vi "HFRR ADV v01.vi"() -> ()   [LabVIEW 2025] (continued)
                w439 = T19."Enabled" ("Disabled")
                n341 = property on="Auto Start Test" class="Bool (strict)"("DisabledEnum"=w439, "TipStrip"=w438) -> ()  [unwired: 2 in, 2 out]
                n342 = property on="RUN" class="Bool (strict)"("DisabledEnum"=w439, "TipStrip"=w438) -> ()  [unwired: 2 in, 2 out]
              }
              frame False {
                w440 = "Enter File Name to Start Test" ("Tip Strip")
                w441 = T19."Disabled and Grayed Out" ("Disabled")
                n343 = property on="Auto Start Test" class="Bool (strict)"("DisabledEnum"=w441, "TipStrip"=w440) -> ()  [unwired: 2 in, 2 out]
                n344 = property on="RUN" class="Bool (strict)"("DisabledEnum"=w441, "TipStrip"=w440) -> ()  [unwired: 2 in, 2 out]
              }
            }
          }
          frame True {
            w442 = "" ("Tip Strip")
            w443 = T19."Enabled" ("Disabled")
            n345 = property on="Auto Start Test" class="Bool (strict)"("DisabledEnum"=w443, "TipStrip"=w442) -> ()  [unwired: 2 in, 2 out]
            n346 = property on="RUN" class="Bool (strict)"("DisabledEnum"=w443, "TipStrip"=w442) -> ()  [unwired: 2 in, 2 out]
          }
        }
      }
      event "RUN": Value Change {
        n347 = event-data() -> ()  [unwired: 1 in, 6 out]
        n348 = local read "RUN"() -> (w445:bool)
        n349 = case shown="False" w445 {
          frame False {
            n350 = flat-sequence {
              frame #0 {
                n351 = local write "START TEMP"(FALSE ("START TEMP")) -> ()
              }
              frame #1 {
                n352 = Wait (ms)(milliseconds to wait=u32 1500) -> ()  [unwired: 1 out]
              }
              frame #2 {
                n353 = local write "Humidity 2"(TRUE ("Humidity")) -> ()
              }
              frame #3 {
                n354 = local write "Due Write"("VC;0") -> ()
              }
              frame #4 {
                n355 = Wait (ms)(milliseconds to wait=u32 1500) -> ()  [unwired: 1 out]
              }
              frame #5 {
                w455 = T19."Enabled" ("Disabled")
                (unwired) T25."Imaging" ("Main Dashboard Buttons")
                (unwired) T21."Adv Scar" ("Main Tab")
                w457 = "" ("FILE")
                n356 = local write "measured_stroke"(0.0 ("measured_stroke")) -> ()
                n357 = local write "Due Write"("VC;0") -> ()
                n358 = local write "FILE"(w457) -> ()
                n359 = local write "Batch Ref Num :"(w457) -> ()
                n360 = local write "Fuel Discription :"(w457) -> ()
                n361 = local write "Main Tab"(T4."Adv Scar" ("Main Tab")) -> ()
                n362 = local write "Remarks :"(w457) -> ()
                n363 = local write "Main Dashboard Buttons"(T1."Imaging" ("Main Dashboard Buttons")) -> ()
                n364 = local write "TEST FILE NAM,E SAVED"(FALSE ("TEST FILE NAM,E SAVED")) -> ()
                n365 = property on="Stroke ( mm )" class="WFChart (strict)"("History Data"=cluster{"y":dbl, dbl, "y":dbl}[] []) -> ()  [unwired: 2 in, 2 out]
                n366 = property on="Auto Start Test" class="Bool (strict)"("Visible"=TRUE) -> ()  [unwired: 2 in, 2 out]
                n367 = property on="FRICVALZ 2" class="Bool (strict)"("DisabledEnum"=w455) -> ()  [unwired: 2 in, 2 out]
                n368 = property on="FRICVALZ 4" class="Bool (strict)"("DisabledEnum"=w455) -> ()  [unwired: 2 in, 2 out]
                n369 = property on="FRICVALZ 3" class="Bool (strict)"("DisabledEnum"=w455) -> ()  [unwired: 2 in, 2 out]
              }
            }
          }
          frame True {
            n370 = stacked-sequence {
              frame #0 {
                n371 = local write "FRICVALZ 4"(TRUE ("FRICVALZ 4")) -> ()
                n372 = local write "Due Write"("DAC;200") -> ()
              }
              frame #1 {
              }
              frame #2 {
              }
              frame #3 {
                n373 = Wait (ms)(milliseconds to wait=u32 1000) -> ()  [unwired: 1 out]
              }
              frame #4 {
                n374 = local write "Due Write"("VC;1") -> ()
              }
              frame #5 {
                n375 = Wait (ms)(milliseconds to wait=u32 1000) -> ()  [unwired: 1 out]
              }
              frame #6 {
                n376 = local write "Due Write"("VC;1") -> ()
              }
              frame #7 {
                n377 = Wait (ms)(milliseconds to wait=u32 1500) -> ()  [unwired: 1 out]
              }
              frame #8 {
                w468 = T19."Disabled" ("Disabled")
                n378 = property on="Auto Start Test" class="Bool (strict)"("Visible"=FALSE) -> ()  [unwired: 2 in, 2 out]
                n379 = local write "START TEMP"(TRUE ("START TEMP")) -> ()
                n380 = property on="FRICVALZ 2" class="Bool (strict)"("DisabledEnum"=w468) -> ()  [unwired: 2 in, 2 out]
                n381 = property on="FRICVALZ 4" class="Bool (strict)"("DisabledEnum"=w468) -> ()  [unwired: 2 in, 2 out]
                n382 = property on="FRICVALZ 3" class="Bool (strict)"("DisabledEnum"=w468) -> ()  [unwired: 2 in, 2 out]
              }
            }
          }
        }
      }
      event "run test Calibration": Value Change {
        n383 = event-data() -> ()  [unwired: 1 in, 6 out]
        n384 = local read "run test Calibration"() -> (w470:bool)
        n385 = case shown="False" w470 {
          frame False {
            n386 = flat-sequence {
              frame #0 {
                n387 = local write "START TEMP"(FALSE ("START TEMP")) -> ()
              }
              frame #1 {
                n388 = Wait (ms)(milliseconds to wait=u32 1500) -> ()  [unwired: 1 out]
              }
              frame #2 {
              }
              frame #3 {
                n389 = local write "Due Write"("VC;0") -> ()
              }
              frame #4 {
                n390 = Wait (ms)(milliseconds to wait=u32 1500) -> ()  [unwired: 1 out]
              }
              frame #5 {
                n391 = local write "Due Write"("VC;0") -> ()
                n392 = property on="Tab Control 6" class="TabCtl (strict)"("Visible"=FALSE) -> ()  [unwired: 2 in, 2 out]
                n393 = local write "Friction Force Calibration Result Tab"(enum32{"Calibration Results", "Page 2"}."Calibration Results" ("Friction Force Calibration Result Tab")) -> ()
                n394 = property on="Friction Force Calibration Result Tab" class="TabCtl (strict)"("Visible"=TRUE) -> ()  [unwired: 2 in, 2 out]
              }
            }
          }
          frame True {
            n395 = flat-sequence {
              frame #0 {
                n396 = local write "Due Write"("VC;1") -> ()
              }
              frame #1 {
                n397 = Wait (ms)(milliseconds to wait=u32 1000) -> ()  [unwired: 1 out]
              }
              frame #2 {
                n398 = local write "Due Write"("VC;1") -> ()
              }
              frame #3 {
                n399 = Wait (ms)(milliseconds to wait=u32 2000) -> ()  [unwired: 1 out]
              }
              frame #4 {
                n400 = local write "START TEMP"(TRUE ("START TEMP")) -> ()
                n401 = property on="Tab Control 6" class="TabCtl (strict)"("Visible"=TRUE) -> ()  [unwired: 2 in, 2 out]
                n402 = local write "Friction Force Calibration Result Tab"(enum32{"Calibration Results", "Page 2"}."Calibration Results" ("Friction Force Calibration Result Tab")) -> ()
              }
            }
          }
        }
      }
      event "Auto": Value Change {
        n403 = event-data() -> ()  [unwired: 1 in, 6 out]
        n404 = stacked-sequence {
          frame #0 {
            n405 = local write "FILE"("") -> ()
          }
          frame #1 {
            n406 = Get Date/Time In Seconds() -> (seconds since 1Jan1904=w491:timestamp)
            n407 = Format Into String(format string="%<%m/%d/%Y %I:%M:%S %p>T", w491) -> (resulting string=w490:string)  [unwired: 2 in, 1 out]
            n408 = local write "FILE"(w490) -> ()
          }
        }
        n409 = local read "Auto"() -> (w488:bool)
        n410 = Not(x=w488) -> (.not. x?=w487:bool)
        n411 = local write "Auto"(w487) -> ()
      }
      event "Auto Start Temp": Value Change {
        n412 = event-data() -> ()  [unwired: 1 in, 6 out]
        n413 = local read "Auto Start Test"() -> (w494:bool)
        n414 = case shown="False" w494 {
          frame False {
            n415 = stacked-sequence {
              frame #0 {
                n416 = local write "START TEMP"(FALSE ("START TEMP")) -> ()
              }
              frame #1 {
                n417 = Wait (ms)(milliseconds to wait=u32 2000) -> ()  [unwired: 1 out]
              }
              frame #2 {
                n418 = local write "Due Write"("VC;0") -> ()
              }
              frame #3 {
                n419 = Wait (ms)(milliseconds to wait=u32 2000) -> ()  [unwired: 1 out]
              }
              frame #4 {
                w505 = T19."Enabled" ("Disabled")
                (unwired) T25."Imaging" ("Main Dashboard Buttons")
                w506 = "" ("FILE")
                n420 = local write "Main Tab"(T4."Adv Scar" ("Main Tab")) -> ()
                n421 = local write "measured_stroke"(0.0 ("measured_stroke")) -> ()
                n422 = local write "Main Dashboard Buttons"(T1."Imaging" ("Main Dashboard Buttons")) -> ()
                n423 = property on="RUN" class="Bool (strict)"("Visible"=TRUE) -> ()  [unwired: 2 in, 2 out]
                n424 = local write "Due Write"("VC;0") -> ()
                n425 = local write "Humidity 2"(TRUE ("Humidity")) -> ()
                n426 = local write "TEST FILE NAM,E SAVED"(FALSE ("TEST FILE NAM,E SAVED")) -> ()
                n427 = local write "Fuel Discription :"(w506) -> ()
                n428 = local write "Batch Ref Num :"(w506) -> ()
                n429 = local write "Remarks :"(w506) -> ()
                n430 = local write "FILE"(w506) -> ()
                n431 = property on="FRICVALZ 2" class="Bool (strict)"("DisabledEnum"=w505) -> ()  [unwired: 2 in, 2 out]
                n432 = property on="FRICVALZ 4" class="Bool (strict)"("DisabledEnum"=w505) -> ()  [unwired: 2 in, 2 out]
                n433 = property on="FRICVALZ 3" class="Bool (strict)"("DisabledEnum"=w505) -> ()  [unwired: 2 in, 2 out]
              }
            }
          }
          frame True {
            n434 = stacked-sequence {
              frame #0 {
                n435 = local write "Due Write"("DAC;200") -> ()
              }
              frame #1 {
                n436 = Wait (ms)(milliseconds to wait=u32 1000) -> ()  [unwired: 1 out]
              }
              frame #2 {
              }
              frame #3 {
              }
              frame #4 {
                n437 = local write "Due Write"("VC;1") -> ()
              }
              frame #5 {
                n438 = Wait (ms)(milliseconds to wait=u32 1000) -> ()  [unwired: 1 out]
              }
              frame #6 {
                n439 = local write "Due Write"("VC;1") -> ()
              }
              frame #7 {
                n440 = Wait (ms)(milliseconds to wait=u32 1500) -> ()  [unwired: 1 out]
              }
              frame #8 {
                w515 = T19."Disabled" ("Disabled")
                n441 = property on="RUN" class="Bool (strict)"("Visible"=FALSE) -> ()  [unwired: 2 in, 2 out]
                n442 = property on="FRICVALZ 2" class="Bool (strict)"("DisabledEnum"=w515) -> ()  [unwired: 2 in, 2 out]
                n443 = property on="FRICVALZ 4" class="Bool (strict)"("DisabledEnum"=w515) -> ()  [unwired: 2 in, 2 out]
                n444 = property on="FRICVALZ 3" class="Bool (strict)"("DisabledEnum"=w515) -> ()  [unwired: 2 in, 2 out]
                "START TEMP" <- TRUE
              }
            }
          }
        }
      }
      event "FILE", "USERNAME", "USER ID": Mouse Enter {
        n445 = event-data() -> ()  [unwired: 1 in, 4 out]
        n446 = dll-call lib="kernel32.dll" fn="Wow64DisableWow64FsRedirection"("OldValue"=0) -> (error out=w522:errorcluster, "OldValue"=w520:i32)  [unwired: 4 in, 1 out]
        n447 = call <vilib>:"System Exec.vi"("run minimized? (F)"=TRUE, "error in (no error)"=w522, "command line"="C:\\Program Files\\Common Files\\Microsoft Shared\\Ink\\TabTip.exe") -> ("error out"=w521:errorcluster)  [unwired: 5 in, 3 out]
        n448 = dll-call lib="kernel32.dll" fn="Wow64EnableWow64FsRedirection"(error in=w521, "OldValue"=w520) -> ()  [unwired: 4 in, 2 out]
      }
      event "EDIT": Value Change {
        n449 = event-data() -> ()  [unwired: 1 in, 6 out]
        n450 = local read "EDIT"() -> (w523:bool)
        n451 = case shown="False" w523 {
          frame False {
            n452 = control-ref of="This VI"() -> (w540:refnum<vi>)
            n453 = property class="VI"(reference=w540) -> (reference out=w531:refnum<vi>, error out=w535:errorcluster, "Panel"=w539:refnum<vi>)  [unwired: 1 in]
            n454 = property class="Pnl"(reference=w539, error in=w535) -> (reference out=w533:refnum<vi>, error out=w536:errorcluster, "Panes[]"=w538:refnum<vi>[])
            n455 = for {
              tunnel: w538 -> [w546] mode=indexing
              tunnel: T24."Always Off" ("Horizontal Scrollbar Visibility") -> [w545]
              tunnel: w536 -> [w542]
              tunnel: [w541] -> w534
              n456 = property class="Pane"(reference=w546, error in=w542, "HorizScrollbarVisibility"=w545) -> (reference out=w543:refnum<vi>, error out=w544:errorcluster)
              n457 = Close Reference(reference=w543, error in (no error)=w544) -> (error out=w541:errorcluster)
            }
            n458 = Close Reference(reference=w533, error in (no error)=w534) -> (error out=w532:errorcluster)
            n459 = Close Reference(reference=w531, error in (no error)=w532) -> (error out=w526:errorcluster)
            "error out 7" <- w526
            n460 = call <vilib>:"Clear Errors.vi"("error in (no error)"=w526) -> ("error out"=w525:errorcluster)  [unwired: 5 in, 1 out]
            n461 = local write "Service Password enable"(FALSE ("Service Password enable")) -> ()
            n462 = call <userlib>:"Fit VI window to Largest Dec.vi"("error in (no error)"=w525, "border spacing (2 px)"=1) -> ("error out"=w530:errorcluster, "dup VI Ref"=w528:refnum<vi>)  [unwired: 4 in]
            n463 = invoke on="Invoke Node" class="VI" method="FP.Run-Time Position.Maximized"(reference=w528, error in=w530) -> (error out=w529:errorcluster)  [unwired: 2 in, 3 out]
            n464 = call <vilib>:"Clear Errors.vi"("error in (no error)"=w529) -> ()  [unwired: 5 in, 2 out]
          }
          frame True {
          }
        }
      }
      event "Heater Button": Value Change {
        n465 = event-data() -> ()  [unwired: 1 in, 6 out]
        n466 = local read "Heater Button"() -> (w547:bool)
        n467 = case shown="True" w547 {
          frame True {
            n468 = stacked-sequence {
              frame #0 {
                n469 = Wait (ms)(milliseconds to wait=u32 1500) -> ()  [unwired: 1 out]
              }
              frame #1 {
                n470 = local read "Set Temp"() -> (w549:dbl)
                n471 = Number To Fractional String(number=w549, precision (6)=i16 2) -> (F-format string=w552:string)  [unwired: 2 in]
                n472 = Concatenate Strings("ST;" ("Command"), w552) -> (w551:string)
                n473 = local write "Due Write"(w551) -> ()
              }
              frame #2 {
                n474 = Wait (ms)(milliseconds to wait=u32 1500) -> ()  [unwired: 1 out]
              }
              frame #3 {
                n475 = local write "Due Write"("HE;1" ("Command")) -> ()
              }
              frame #4 {
                n476 = Wait (ms)(milliseconds to wait=u32 1500) -> ()  [unwired: 1 out]
              }
              frame #5 {
                n477 = stacked-sequence {
                  frame #0 {
                    n478 = Wait (ms)(milliseconds to wait=u32 1500) -> ()  [unwired: 1 out]
                  }
                  frame #1 {
                    n479 = local read "Set Temp"() -> (w558:dbl)
                    n480 = Number To Fractional String(number=w558, precision (6)=i16 2) -> (F-format string=w561:string)  [unwired: 2 in]
                    n481 = Concatenate Strings("ST;" ("Command"), w561) -> (w560:string)
                    n482 = local write "Due Write"(w560) -> ()
                  }
                  frame #2 {
                    n483 = Wait (ms)(milliseconds to wait=u32 1500) -> ()  [unwired: 1 out]
                  }
                  frame #3 {
                    n484 = local write "Due Write"("HE;1" ("Command")) -> ()
                  }
                  frame #4 {
                    n485 = Wait (ms)(milliseconds to wait=u32 1500) -> ()  [unwired: 1 out]
                  }
                }
              }
            }
          }
          frame False {
            n486 = stacked-sequence {
              frame #0 {
                n487 = Wait (ms)(milliseconds to wait=u32 1500) -> ()  [unwired: 1 out]
              }
              frame #1 {
                n488 = Concatenate Strings("ST;" ("Command"), "0" ("string")) -> (w568:string)
                n489 = local write "Due Write"(w568) -> ()
              }
              frame #2 {
                n490 = Wait (ms)(milliseconds to wait=u32 1500) -> ()  [unwired: 1 out]
              }
              frame #3 {
                n491 = local write "Due Write"("HE;0" ("Command")) -> ()
              }
              frame #4 {
                n492 = Wait (ms)(milliseconds to wait=u32 1500) -> ()  [unwired: 1 out]
              }
            }
          }
        }
      }
      event "Headen Service Button": Value Change {
        n493 = event-data() -> ()  [unwired: 1 in, 6 out]
        n494 = local read "Headen Service Button"() -> (w573:bool)
        n495 = case shown="True" w573 {
          frame False {
            n496 = property on="Password 3" class="Clust (strict)"("Visible"=FALSE) -> ()  [unwired: 2 in, 2 out]
            n497 = property on="Service Password Log" class="Str"("Visible"=FALSE) -> ()  [unwired: 2 in, 2 out]
          }
          frame True {
            n498 = flat-sequence {
              tunnel: [w579] -> w576
              tunnel: w576 -> [w580]
              frame #0 {
                n499 = property on="Password 3" class="Clust (strict)"("Visible"=TRUE) -> ()  [unwired: 2 in, 2 out]
                n500 = property on="Service Password Log" class="Str"("Visible"=TRUE) -> ()  [unwired: 2 in, 2 out]
              }
              frame #1 {
                n501 = call "DIALOG BOX HFRR ADV.vi"() -> ("Continue"=w579:bool)  [unwired: 8 in, 2 out]
              }
              frame #2 {
                n502 = case shown="True" w580 {
                  frame True {
                    n503 = property on="Password 3" class="Clust (strict)"("Visible"=TRUE) -> ()  [unwired: 2 in, 2 out]
                    n504 = property on="Service Password Log" class="Str"("Visible"=TRUE) -> ()  [unwired: 2 in, 2 out]
                  }
                  frame False {
                    n505 = property on="Password 3" class="Clust (strict)"("Visible"=FALSE) -> ()  [unwired: 2 in, 2 out]
                    n506 = property on="Service Password Log" class="Str"("Visible"=FALSE) -> ()  [unwired: 2 in, 2 out]
                  }
                }
              }
            }
          }
        }
      }
      event "Password 3.Service Password": Value Change {
        n507 = event-data() -> ()  [unwired: 1 in, 6 out]
        n508 = Unbundle By Name("Password 3") -> ("Service Password"=w587:string)
        n509 = call <vilib>:"Trim Whitespace.vi"("string"=w587) -> ("trimmed string"=w585:string)  [unwired: 1 in]
        n510 = Equal?(x=w585, y="Service@123") -> (x = y?=w586:bool)
        n511 = case shown="True" w586 {
          selector: w586 -> [w591 w594]
          frame False {
            w590 = FALSE
            n512 = local write "Service Password enable"(w591) -> ()
            n513 = property on="Service Password Log" class="Str"("Visible"=TRUE) -> ()  [unwired: 2 in, 2 out]
            n514 = property on="Service Left" class="Bool (strict)"("Visible"=w590) -> ()  [unwired: 2 in, 2 out]
            n515 = property on="Service Right" class="Bool (strict)"("Visible"=w590) -> ()  [unwired: 2 in, 2 out]
            n516 = property on="Service Bottom" class="Bool (strict)"("Visible"=w590) -> ()  [unwired: 2 in, 2 out]
          }
          frame True {
            w593 = TRUE
            n517 = property on="Service Password Log" class="Str"("Visible"=FALSE) -> ()  [unwired: 2 in, 2 out]
            n518 = property on="Service Left" class="Bool (strict)"("Visible"=w593) -> ()  [unwired: 2 in, 2 out]
            n519 = property on="Service Right" class="Bool (strict)"("Visible"=w593) -> ()  [unwired: 2 in, 2 out]
            n520 = property on="Service Bottom" class="Bool (strict)"("Visible"=w593) -> ()  [unwired: 2 in, 2 out]
            "Service Password enable" <- w594
          }
        }
      }
      event "Sign In": Value Change {
        w596 = FALSE ("Visible")
        n521 = event-data() -> ()  [unwired: 1 in, 6 out]
        n522 = property on="About" class="Clust (strict)"("Visible"=w596) -> ()  [unwired: 2 in, 2 out]
        n523 = property on="Password 3" class="Clust (strict)"("Visible"=w596) -> ()  [unwired: 2 in, 2 out]
        n524 = property on="Service Password Log" class="Str"("Visible"=FALSE) -> ()  [unwired: 2 in, 2 out]
      }
      event "Info": Value Change {
        n525 = event-data() -> ()  [unwired: 1 in, 6 out]
        n526 = local read "Operating System"() -> (w601:string)
        n527 = local read "Firmware Version"() -> (w602:string)
        n528 = local read "Instrument Serial"() -> (w600:string)
        n529 = local read "Workorder"() -> (w604:string)
        n530 = local write "Info"(FALSE) -> ()
        n531 = local read "Runtime"() -> (w603:string)
        n532 = local read "Version"() -> (w605:string)
        n533 = local read "version"() -> (w606:string)
        n534 = Insert Into Array(array=string[] [], new element #1=w606, new element #2=w605, new element #3=w604, new element #4=w603, new element #5=w602, new element #6=w601, new element #7=w600) -> (w599:string[])  [unwired: 1 in]
        n535 = call "ABOUT SCREEN ADV NEW.vi"("Array"=w599) -> ()  [unwired: 10 in, 1 out]
      }
      event "Calibration": Value Change {
        n536 = event-data() -> ()  [unwired: 1 in, 6 out]
        n537 = local read "Calibration"() -> (w609:bool)
        n538 = case shown="False" w609 {
          frame False {
            n539 = property on="Calibration 2" class="TabCtl (strict)"("Visible"=FALSE) -> ()  [unwired: 2 in, 2 out]
            n540 = local write "Cal Password"("" ("Cal Password")) -> ()
          }
          frame True {
            n541 = property on="Calibration 2" class="TabCtl (strict)"("Visible"=TRUE) -> ()  [unwired: 2 in, 2 out]
            n542 = local write "Cal Password"("" ("Cal Password")) -> ()
          }
        }
        n543 = property on="Wrong Password" class="Str"("Visible"=FALSE) -> ()  [unwired: 2 in, 2 out]
      }
      event "Cal Password": Value Change {
        n544 = event-data() -> ()  [unwired: 1 in, 6 out]
        n545 = local read "Cal Password"() -> (w617:string)
        n546 = call <vilib>:"Trim Whitespace.vi"("string"=w617) -> ("trimmed string"=w616:string)  [unwired: 1 in]
        n547 = Equal?(x=w616, y="Cal@321") -> (x = y?=w614:bool)
        n548 = case shown="True" w614 {
          frame False {
            n549 = property on="Wrong Password" class="Str"("Visible"=TRUE) -> ()  [unwired: 2 in, 2 out]
          }
          frame True {
            n550 = property on="Wrong Password" class="Str"("Visible"=FALSE) -> ()  [unwired: 2 in, 2 out]
            n551 = local write "Main Tab"(T4."About" ("Main Tab")) -> ()
            n552 = local write "Cal Password"("" ("Cal Password")) -> ()
            n553 = local write "Main Dashboard Buttons"(T1."About" ("Main Dashboard Buttons")) -> ()
            n554 = property on="Calibration 2" class="TabCtl (strict)"("Visible"=FALSE) -> ()  [unwired: 2 in, 2 out]
            n555 = local write "Calibration"(FALSE ("Calibration")) -> ()
          }
        }
      }
      event "Calibration Selection": Value Change {
        n556 = event-data() -> ()  [unwired: 1 in, 6 out]
        n557 = local read "Calibration Selection"() -> (w626:T10)
        n558 = case shown="\"Stroke Calibration\"" w626 {
          tunnel: [T9."Stroke" ("Main Calibration Tab") T9."Friction" ("Main Calibration Tab") T9."Main" ("Main Calibration Tab") T9."Temperature" ("Main Calibration Tab")] -> w625
          frame "Stroke Calibration" {
          }
          frame "Friction Force Calibration" {
          }
          frame Default {
          }
          frame "Temperature Calibration" {
          }
        }
        n559 = local write "Main Calibration Tab"(w625) -> ()
      }
      event "Back Stroke": Value Change {
        n560 = event-data() -> ()  [unwired: 1 in, 6 out]
        n561 = local write "Main Stroke Tab"(T11."Step 1" ("Main Stroke Tab")) -> ()
        n562 = local write "Main Calibration Tab"(T9."Main" ("Main Calibration Tab")) -> ()
        n563 = local write "Back Stroke"(FALSE ("Back Stroke")) -> ()
        n564 = local write "Calibration Selection"(T10."Default" ("Calibration Selection")) -> ()
      }
      event "Step 2 Back": Value Change {
        n565 = event-data() -> ()  [unwired: 1 in, 6 out]
        n566 = local write "Main Stroke Tab"(T11."Step 1" ("Main Stroke Tab")) -> ()
        n567 = local write "Step 2 Back"(FALSE ("Back Stroke")) -> ()
        n568 = local write "Calibration Selection"(T10."Default" ("Calibration Selection")) -> ()
      }
      event "Step 3 Back": Value Change {
        n569 = event-data() -> ()  [unwired: 1 in, 6 out]
        n570 = local write "Main Stroke Tab"(T11."Step 2" ("Main Stroke Tab")) -> ()
        n571 = local write "Step 3 Back"(FALSE ("Back Stroke")) -> ()
        n572 = local write "Calibration Selection"(T10."Default" ("Calibration Selection")) -> ()
      }
      event "Step 4 Back": Value Change {
        n573 = event-data() -> ()  [unwired: 1 in, 6 out]
        n574 = local write "Main Stroke Tab"(T11."Step 3" ("Main Stroke Tab")) -> ()
        n575 = local write "Step 4 Back"(FALSE ("Back Stroke")) -> ()
        n576 = local write "Calibration Selection"(T10."Default" ("Calibration Selection")) -> ()
      }
      event "Step 5 Back": Value Change {
        n577 = event-data() -> ()  [unwired: 1 in, 6 out]
        n578 = local write "Main Stroke Tab"(T11."Step 4" ("Main Stroke Tab")) -> ()
        n579 = local write "Step 5 Back"(FALSE ("Back Stroke")) -> ()
        n580 = local write "Calibration Selection"(T10."Default" ("Calibration Selection")) -> ()
      }
      event "Step 6 Back": Value Change {
        n581 = event-data() -> ()  [unwired: 1 in, 6 out]
        n582 = local write "Main Stroke Tab"(T11."Step 5" ("Main Stroke Tab")) -> ()
        n583 = local write "Step 6 Back"(FALSE ("Back Stroke")) -> ()
        n584 = local write "Calibration Selection"(T10."Default" ("Calibration Selection")) -> ()
      }
      event "Back Stroke step 7": Value Change {
        n585 = event-data() -> ()  [unwired: 1 in, 6 out]
        n586 = local write "Main Stroke Tab"(T11."Step 5" ("Main Stroke Tab")) -> ()
        n587 = local write "Back Stroke step 7"(FALSE ("Back Stroke")) -> ()
        n588 = local write "Calibration Selection"(T10."Default" ("Calibration Selection")) -> ()
      }
      event "Back Stroke step 8": Value Change {
        n589 = event-data() -> ()  [unwired: 1 in, 6 out]
        n590 = local write "Main Stroke Tab"(T11."Step 7" ("Main Stroke Tab")) -> ()
        n591 = local write "Back Stroke step 8"(FALSE ("Back Stroke")) -> ()
        n592 = local write "Calibration Selection"(T10."Default" ("Calibration Selection")) -> ()
      }
      event "Back Stroke 8": Value Change {
        n593 = event-data() -> ()  [unwired: 1 in, 6 out]
        n594 = local write "MOVE CARRIAGE TO"(1.0 ("MOVE CARRIAGE TO")) -> ()
        n595 = local write "Main Stroke Tab"(T11."Step 1" ("Main Stroke Tab")) -> ()
        n596 = local write "Calibration Selection"(T10."Default" ("Calibration Selection")) -> ()
        n597 = local write "Back Stroke 8"(FALSE ("Back Stroke 8")) -> ()
      }
      event "Continue Stroke": Value Change {
        n598 = event-data() -> ()  [unwired: 1 in, 6 out]
        n599 = local write "Main Stroke Tab"(T11."Step 2" ("Main Stroke Tab")) -> ()
        n600 = local write "Continue Stroke"(FALSE ("Continue Stroke")) -> ()
      }
      event "Continue Stroke step 2": Value Change {
        n601 = event-data() -> ()  [unwired: 1 in, 6 out]
        n602 = local write "Main Stroke Tab"(T11."Step 3" ("Main Stroke Tab")) -> ()
        n603 = local write "Continue Stroke step 2"(FALSE ("Continue Stroke")) -> ()
      }
      event "Continue Stroke step 3": Value Change {
        n604 = event-data() -> ()  [unwired: 1 in, 6 out]
        n605 = local write "Main Stroke Tab"(T11."Step 4" ("Main Stroke Tab")) -> ()
        n606 = local write "Continue Stroke step 3"(FALSE ("Continue Stroke")) -> ()
      }
      event "Continue Stroke step 4": Value Change {
        n607 = event-data() -> ()  [unwired: 1 in, 6 out]
        n608 = local write "Main Stroke Tab"(T11."Step 5" ("Main Stroke Tab")) -> ()
        n609 = local write "Continue Stroke step 4"(FALSE ("Continue Stroke")) -> ()
      }
      event "Continue Stroke step 5": Value Change {
        n610 = event-data() -> ()  [unwired: 1 in, 6 out]
        n611 = local write "Main Stroke Tab"(T11."Step 7" ("Main Stroke Tab")) -> ()
        n612 = local write "Continue Stroke step 5"(FALSE ("Continue Stroke")) -> ()
      }
      event "Continue Stroke step 6": Value Change {
        n613 = event-data() -> ()  [unwired: 1 in, 6 out]
        n614 = local write "Main Stroke Tab"(T11."Step 7" ("Main Stroke Tab")) -> ()
        n615 = local write "Continue Stroke step 6"(FALSE ("Continue Stroke")) -> ()
      }
      event "Continue Stroke step 7": Value Change {
        w674 = FALSE ("0.2mm")
        n616 = event-data() -> ()  [unwired: 1 in, 6 out]
        n617 = local write "0.4 mm"(w674) -> ()
        n618 = local write "0.6 mm"(w674) -> ()
        n619 = local write "1.0 mm"(w674) -> ()
        n620 = local write "1.2 mm"(w674) -> ()
        n621 = local write "0.2 2"(w674) -> ()
        n622 = local write "0.4 2"(w674) -> ()
        n623 = local write "0.6 2"(w674) -> ()
        n624 = local write "0.8 2"(w674) -> ()
        n625 = local write "1.0 2"(w674) -> ()
        n626 = local write "1.2"(w674) -> ()
        n627 = local write "0.2mm"(w674) -> ()
        n628 = local write "0.8mm"(w674) -> ()
        n629 = local write "Main Stroke Tab"(T11."Step 8" ("Main Stroke Tab")) -> ()
        n630 = local write "Continue Stroke step 7"(FALSE ("Continue Stroke")) -> ()
        n631 = local write "Stroke Test Complete"(T12."Test Progress" ("Stroke Test Complete")) -> ()
        "Position Measurment Temp" <- 4.0 ("Position Measurment Temp")
        "Calibration Tare" <- TRUE ("Calibration Tare")
        "MOVE CARRIAGE TO" <- 1.0 ("MOVE CARRIAGE TO")
      }
      event "Continue Stroke step 8": Value Change {
        n632 = event-data() -> ()  [unwired: 1 in, 6 out]
        n633 = local read "LVDT STROKE  Calibration"() -> (w679:dbl)
        n634 = local read "Position Measurment Temp"() -> (w680:dbl)
        n635 = case shown="7" w680 {
          selector: w680 -> [w685 w690 w695 w700 _ w708 w711 w712]
          tunnel: w679 -> [w681 w686 w691 w696 w702 w705 _ _]
          frame 0, Default {
            w683 = TRUE ("0.2mm")
            n636 = Increment(x=w685) -> (x+1=w684:i32)
            n637 = local write "Position Measurment Temp"(w684) -> ()
            n638 = local write "0.2mm"(w683) -> ()
            n639 = local write "0.2 2"(w683) -> ()
            n640 = local write "MOVE CARRIAGE TO"(1.0 ("MOVE CARRIAGE TO")) -> ()
            "Calibration 0.2" <- w681
          }
          frame 1 {
            w688 = TRUE ("0.4 mm")
            n641 = Increment(x=w690) -> (x+1=w689:i32)
            n642 = local write "Calibration 0.4"(w686) -> ()
            n643 = local write "Position Measurment Temp"(w689) -> ()
            n644 = local write "0.4 mm"(w688) -> ()
            n645 = local write "MOVE CARRIAGE TO"(0.6 ("MOVE CARRIAGE TO")) -> ()
            n646 = local write "0.4 2"(w688) -> ()
          }
          frame 2 {
            w693 = TRUE ("0.6 mm")
            n647 = Increment(x=w695) -> (x+1=w694:i32)
            n648 = local write "Calibration 0.6"(w691) -> ()
            n649 = local write "Position Measurment Temp"(w694) -> ()
            n650 = local write "0.6 2"(w693) -> ()
            n651 = local write "0.6 mm"(w693) -> ()
            n652 = local write "MOVE CARRIAGE TO"(0.8 ("MOVE CARRIAGE TO")) -> ()
          }
          frame 3 {
            w697 = TRUE ("0.6 mm")
            n653 = Increment(x=w700) -> (x+1=w699:i32)
            n654 = local write "Position Measurment Temp"(w699) -> ()
            n655 = local write "MOVE CARRIAGE TO"(1.0 ("MOVE CARRIAGE TO")) -> ()
            n656 = local write "0.8mm"(w697) -> ()
            n657 = local write "0.8 2"(w697) -> ()
            "Calibration 0.8" <- w696
          }
          frame 4 {
            w703 = TRUE ("0.6 mm")
            n658 = local write "Position Measurment Temp"(6.0 ("Position Measurment Temp")) -> ()
            n659 = local write "MOVE CARRIAGE TO"(1.0 ("MOVE CARRIAGE TO")) -> ()
            n660 = local write "1.0 mm"(w703) -> ()
            n661 = local write "1.0 2"(w703) -> ()
            "Calibration 1.0" <- w702
          }
          frame 5 {
            w706 = TRUE ("0.6 mm")
            n662 = Increment(x=w708) -> (x+1=w707:i32)
            n663 = local write "Position Measurment Temp"(w707) -> ()
            n664 = local write "1.2 mm"(w706) -> ()
            n665 = local write "1.2"(w706) -> ()
            "Calibration 1.2" <- w705
          }
          frame 6 {
            n666 = Increment(x=w711) -> (x+1=w710:i32)
            n667 = local write "Position Measurment Temp"(w710) -> ()
            n668 = local write "Stroke Test Complete"(T12."Stroke Points Completed" ("Stroke Test Complete")) -> ()
          }
          frame 7 {
            n669 = stacked-sequence {
              tunnel: w712 -> [w713 _ _]
              frame #0 {
                n670 = Increment(x=w713) -> (x+1=w714:i32)
                n671 = local write "Main Stroke Tab"(T11."Step 9" ("Main Stroke Tab")) -> ()
                n672 = local write "Position Measurment Temp"(w714) -> ()
                n673 = Insert Into Array(array=dbl[] [], new element #1=0.2 ("new element/subarray"), new element #2=0.4 ("new element/subarray"), new element #3=0.6 ("new element/subarray"), new element #4=0.8 ("new element/subarray"), new element #5=1.0 ("new element/subarray"), new element #6=1.2 ("new element/subarray")) -> (→"1D stroke":dbl[])  [unwired: 1 in]
                n674 = local read "Calibration 0.2"() -> (w721:dbl)
                n675 = local read "Calibration 0.4"() -> (w720:dbl)
                n676 = local read "Calibration 0.6"() -> (w719:dbl)
                n677 = local read "Calibration 0.8"() -> (w718:dbl)
                n678 = local read "Calibration 1.0"() -> (w717:dbl)
                n679 = local read "Calibration 1.2"() -> (w716:dbl)
                n680 = Insert Into Array(array=dbl[] [], new element #1=w721, new element #2=w720, new element #3=w719, new element #4=w718, new element #5=w717, new element #6=w716) -> (→"Calibrated Voltage Value":dbl[])  [unwired: 1 in]
              }
              frame #1 {
                n681 = local read "calibration values"() -> (w744:dbl[])
                n682 = local read "Calibrated Voltage Value"() -> (w746:dbl[])
                n683 = Index Array(array=w744, index #1=1 ("index"), index #2=3 ("index"), index #3=5 ("index"), index #4=7 ("index"), index #5=9 ("index"), index #6=11 ("index")) -> (element #1=w737:dbl, element #2=w736:dbl, element #3=w735:dbl, element #4=w734:dbl, element #5=w733:dbl, element #6=w732:dbl)
                n684 = local read "1D stroke"() -> (w747:dbl[])
                n685 = for {
                  tunnel: [w756] -> w745 mode=indexing
                  tunnel: w747 -> [w755] mode=indexing
                  tunnel: w746 -> [w754] mode=indexing
                  tunnel: w737 -> [w753]
                  tunnel: w736 -> [w752]
                  tunnel: w735 -> [w751]
                  tunnel: w734 -> [w750]
                  tunnel: w733 -> [w749]
                  tunnel: w732 -> [w748]
                  n686 = formula code="if (stroke == 0.2)\n{\n    if ((voltage >= REF_02 - 0.2) && (voltage <= REF_02 + 0.2))\n        status = 1;\n    else\n        status = 0;\n}\nelse if (stroke == 0.4)\n{\n    if ((voltage >= REF_04 - 0.2) && (voltage <= REF_04 + 0.2))\n        status = 1;\n    else\n        status = 0;\n}\nelse if (stroke == 0.6)\n{\n    if ((voltage >= REF_06 - 0.2) && (voltage <= REF_06 + 0.2))\n        status = 1;\n    else\n        status = 0;\n}\nelse if (stroke == 0.8)\n{\n    if ((voltage >= REF_08 - 0.2) && (voltage <= REF_08 + 0.2))\n        status = 1;\n    else\n        status = 0;\n}\nelse if (stroke == 1.0)\n{\n    if ((voltage >= REF_10 - 1) && (voltage <= REF_10 + 1))\n        status = 1;\n    else\n        status = 0;\n}\nelse if (stroke == 1.2)\n{\n    if ((voltage >= REF_12 - 0.2) && (voltage <= REF_12 + 0.2))\n        status = 1;\n    else\n        status = 0;\n}\nelse\n{\n    status = 0;\n}"("stroke"=w755, "voltage"=w754, "REF_02"=w753, "REF_04"=w752, "REF_06"=w751, "REF_08"=w750, "REF_10"=w749, "REF_12"=w748) -> ("status"=w756:dbl)
                }
                "Status" <- w745
              }
              frame #2 {
                w763 = 1.0
                n687 = local read "Status"() -> (w770:dbl[])
                n688 = Index Array(array=w770) -> (element #1=w769:dbl, element #2=w768:dbl, element #3=w767:dbl, element #4=w766:dbl, element #5=w765:dbl, element #6=w764:dbl)  [unwired: 6 in]
                n689 = Equal?(x=w768, y=w763) -> (x = y?=w761:bool)
                n690 = Equal?(x=w767, y=w763) -> (x = y?=w760:bool)
                n691 = Equal?(x=w766, y=w763) -> (x = y?=w759:bool)
                n692 = Equal?(x=w765, y=w763) -> (x = y?=w758:bool)
                n693 = Equal?(x=w764, y=w763) -> (x = y?=w757:bool)
                n694 = Equal?(x=w769, y=w763) -> (x = y?=w762:bool)
                n695 = case shown="True" w762 {
                  selector: w762 -> [w781 w782]
                  frame True {
                    n696 = local write "Point 1 - 0.2 mm"(w781) -> ()
                    n697 = property on="Point 1 - 0.2 mm" class="Bool"("Caption.Visible"=w781) -> ()  [unwired: 2 in, 2 out]
                  }
                  frame False {
                    n698 = local write "Point 1 - 0.2 mm"(w782) -> ()
                    n699 = property on="Point 1 - 0.2 mm" class="Bool"("Caption.Visible"=w782) -> ()  [unwired: 2 in, 2 out]
                  }
                }
                n700 = case shown="True" w761 {
                  selector: w761 -> [w779 w780]
                  frame True {
                    n701 = local write "Point 2 - 0.4 mm"(w779) -> ()
                    n702 = property on="Point 2 - 0.4 mm" class="Bool"("Caption.Visible"=w779) -> ()  [unwired: 2 in, 2 out]
                  }
                  frame False {
                    n703 = local write "Point 2 - 0.4 mm"(w780) -> ()
                    n704 = property on="Point 2 - 0.4 mm" class="Bool"("Caption.Visible"=w780) -> ()  [unwired: 2 in, 2 out]
                  }
                }
                n705 = case shown="True" w758 {
                  selector: w758 -> [w773 w774]
                  frame True {
                    n706 = local write "Point 5 - 1.0 mm"(w773) -> ()
                    n707 = property on="Point 5 - 1.0 mm" class="Bool"("Caption.Visible"=w773) -> ()  [unwired: 2 in, 2 out]
                  }
                  frame False {
                    n708 = local write "Point 5 - 1.0 mm"(w774) -> ()
                    n709 = property on="Point 5 - 1.0 mm" class="Bool"("Caption.Visible"=w774) -> ()  [unwired: 2 in, 2 out]
                  }
                }
                n710 = case shown="True" w760 {
                  selector: w760 -> [w777 w778]
                  frame True {
                    n711 = local write "Point 3 - 0.6 mm"(w777) -> ()
                    n712 = property on="Point 3 - 0.6 mm" class="Bool"("Caption.Visible"=w777) -> ()  [unwired: 2 in, 2 out]
                  }
                  frame False {
                    n713 = local write "Point 3 - 0.6 mm"(w778) -> ()
                    n714 = property on="Point 3 - 0.6 mm" class="Bool"("Caption.Visible"=w778) -> ()  [unwired: 2 in, 2 out]
                  }
                }
                n715 = case shown="True" w759 {
                  selector: w759 -> [w775 w776]
                  frame True {
                    n716 = local write "Point 4 - 0.8 mm"(w775) -> ()
                    n717 = property on="Point 4 - 0.8 mm" class="Bool"("Caption.Visible"=w775) -> ()  [unwired: 2 in, 2 out]
                  }
                  frame False {
                    n718 = local write "Point 4 - 0.8 mm"(w776) -> ()
                    n719 = property on="Point 4 - 0.8 mm" class="Bool"("Caption.Visible"=w776) -> ()  [unwired: 2 in, 2 out]
                  }
                }
                n720 = case shown="True" w757 {
                  selector: w757 -> [w771 w772]
                  frame True {
                    n721 = local write "Point 6 - 1.2 mm"(w771) -> ()
                    n722 = property on="Point 6 - 1.2 mm" class="Bool"("Caption.Visible"=w771) -> ()  [unwired: 2 in, 2 out]
                  }
                  frame False {
                    n723 = local write "Point 6 - 1.2 mm"(w772) -> ()
                    n724 = property on="Point 6 - 1.2 mm" class="Bool"("Caption.Visible"=w772) -> ()  [unwired: 2 in, 2 out]
                  }
                }
              }
            }
          }
        }
      }
      event "Accept & Save": Value Change {
        n725 = event-data() -> ()  [unwired: 1 in, 6 out]
        n726 = flat-sequence {
          frame #0 {
            n727 = Get Date/Time In Seconds() -> (seconds since 1Jan1904=w785:timestamp)
            n728 = Format Into String(format string="%<%m/%d/%Y %I:%M:%S %p>T", w785) -> (resulting string=w783:string)  [unwired: 2 in, 1 out]
            n729 = local write "STROKE CALIBRATION"(w783) -> ()
          }
          frame #1 {
            n730 = local write "Save Button"(TRUE ("Save Button")) -> ()
          }
          frame #2 {
            n731 = local write "MOVE CARRIAGE TO"(1.0 ("MOVE CARRIAGE TO")) -> ()
            n732 = local write "Main Calibration Tab"(T9."Main" ("Main Calibration Tab")) -> ()
            n733 = local write "Main Stroke Tab"(T11."Step 1" ("Main Stroke Tab")) -> ()
            n734 = local write "Calibration Selection"(T10."Default" ("Calibration Selection")) -> ()
            n735 = local write "Back Stroke 8"(FALSE ("Back Stroke 8")) -> ()
          }
        }
      }
      event "TEMPERATURE STEP Back 1", "TEMPERATURE STEP Back air Temp": Value Change {
        n736 = event-data() -> ()  [unwired: 1 in, 6 out]
        n737 = stacked-sequence {
          frame #0 {
            n738 = local write "Main Calibration Tab"(T9."Main" ("Main Calibration Tab")) -> ()
            n739 = local write "Tab Control 4"(T14."Main" ("Tab Control 4")) -> ()
            n740 = local write "Temperature Selection"(T15."Default" ("Temperature Selection")) -> ()
          }
          frame #1 {
            n741 = Wait (ms)(milliseconds to wait=u32 1000) -> ()  [unwired: 1 out]
            n742 = local write "Calibration Selection"(T10."Default" ("Calibration Selection")) -> ()
          }
          frame #2 {
            n743 = local write "Due Write"("CAL;END" ("Command")) -> ()
          }
          frame #3 {
            n744 = Wait (ms)(milliseconds to wait=u32 2000) -> ()  [unwired: 1 out]
          }
          frame #4 {
            n745 = local write "Due Write"("CAL;END" ("Command")) -> ()
          }
        }
      }
      event "Temperature Continue Step 1": Value Change {
        n746 = event-data() -> ()  [unwired: 1 in, 6 out]
        n747 = stacked-sequence {
          frame #0 {
            n748 = Wait (ms)(milliseconds to wait=u32 1000) -> ()  [unwired: 1 out]
          }
          frame #1 {
            n749 = local write "Due Write"("CAL;START" ("Command")) -> ()
          }
          frame #2 {
            n750 = Wait (ms)(milliseconds to wait=u32 500) -> ()  [unwired: 1 out]
          }
          frame #3 {
            n751 = local write "Due Write"("CAL;START" ("Command")) -> ()
          }
          frame #4 {
            n752 = Wait (ms)(milliseconds to wait=u32 1000) -> ()  [unwired: 1 out]
          }
          frame #5 {
          }
          frame #6 {
          }
          frame #7 {
          }
          frame #8 {
            n753 = local write "Tab Control 4"(T14."Step 2" ("Tab Control 4")) -> ()
          }
        }
      }
      event "Temperature Continue Step air Step 1": Value Change {
        n754 = event-data() -> ()  [unwired: 1 in, 6 out]
        n755 = stacked-sequence {
          frame #0 {
            n756 = Wait (ms)(milliseconds to wait=u32 1000) -> ()  [unwired: 1 out]
          }
          frame #1 {
            n757 = local write "Due Write"("CAL;START" ("Command")) -> ()
          }
          frame #2 {
            n758 = Wait (ms)(milliseconds to wait=u32 1000) -> ()  [unwired: 1 out]
          }
          frame #3 {
            n759 = local write "Due Write"("CAL;START" ("Command")) -> ()
          }
          frame #4 {
          }
          frame #5 {
          }
          frame #6 {
          }
          frame #7 {
          }
          frame #8 {
            n760 = local write "Tab Control 4"(T14."Air Step 2" ("Tab Control 4")) -> ()
          }
        }
      }
      event "Temperature Selection": Value Change {
        n761 = event-data() -> ()  [unwired: 1 in, 6 out]
        n762 = local read "Temperature Selection"() -> (w811:T15)
        n763 = case shown="\"Sample Temperature\"" w811 {
          frame "Air Temperature" {
            n764 = local write "Tab Control 4"(T14."Air Step 1" ("Tab Control 4")) -> ()
          }
          frame "Sample Temperature" {
            n765 = local write "Tab Control 4"(T14."Step 1" ("Tab Control 4")) -> ()
          }
          frame "Default", Default {
          }
        }
      }
      event "Temperature Continue Step 2": Value Change {
        n766 = event-data() -> ()  [unwired: 1 in, 6 out]
        n767 = stacked-sequence {
          frame #0 {
            n768 = stacked-sequence {
              frame #0 {
                n769 = Wait (ms)(milliseconds to wait=u32 1500) -> ()  [unwired: 1 out]
              }
              frame #1 {
                # "CAL;A1;<true_T>"
                n770 = local read "Sensor value"() -> (→"Sample 0deg temp":dbl)
                n771 = local write "Due Write"("CAL;A1;0" ("Command")) -> ()
              }
              frame #2 {
                n772 = Wait (ms)(milliseconds to wait=u32 1500) -> ()  [unwired: 1 out]
              }
              frame #3 {
                # "CAL;A1;<true_T>"
                n773 = local write "Due Write"("CAL;A1;0" ("Command")) -> ()
              }
              frame #4 {
              }
            }
          }
          frame #1 {
            n774 = local write "Tab Control 4"(T14."Step 3" ("Tab Control 4")) -> ()
          }
        }
      }
      event "Temperature Continue Air Step 2": Value Change {
        n775 = event-data() -> ()  [unwired: 1 in, 6 out]
        n776 = stacked-sequence {
          frame #0 {
            n777 = stacked-sequence {
              frame #0 {
                n778 = Wait (ms)(milliseconds to wait=u32 1000) -> ()  [unwired: 1 out]
              }
              frame #1 {
                # "CAL;A1;<true_T>"
                n779 = local write "Due Write"("CAL;A1;0" ("Command")) -> ()
              }
              frame #2 {
                n780 = Wait (ms)(milliseconds to wait=u32 1000) -> ()  [unwired: 1 out]
              }
              frame #3 {
                # "CAL;A1;<true_T>"
                n781 = local write "Due Write"("CAL;A1;0" ("Command")) -> ()
              }
              frame #4 {
                n782 = local read "Sensor value"() -> (→"Air 0deg temp":dbl)
              }
            }
          }
          frame #1 {
            n783 = local write "Tab Control 4"(T14."Air Step 3" ("Tab Control 4")) -> ()
          }
        }
      }
      event "Temperature Continue Step 3": Value Change {
        n784 = event-data() -> ()  [unwired: 1 in, 6 out]
        n785 = stacked-sequence {
          frame #0 {
            n786 = stacked-sequence {
              frame #0 {
                n787 = Wait (ms)(milliseconds to wait=u32 1500) -> ()  [unwired: 1 out]
              }
              frame #1 {
              }
              frame #2 {
              }
              frame #3 {
                # "CAL;A1;<true_T>"
                n788 = local write "Due Write"("CAL;A1;60" ("Command")) -> ()
              }
              frame #4 {
                n789 = Wait (ms)(milliseconds to wait=u32 1000) -> ()  [unwired: 1 out]
              }
              frame #5 {
                # "CAL;A1;<true_T>"
                n790 = local read "Sensor value"() -> (→"Sample 60deg temp":dbl)
                n791 = local write "Due Write"("CAL;A1;60" ("Command")) -> ()
              }
            }
          }
          frame #1 {
            w831 = 0.0
            w832 = 60.0
            n792 = local read "Sample 0deg temp"() -> (w842:dbl)
            n793 = local read "Sample 60deg temp"() -> (w841:dbl)
            n794 = Add(x=w832, y="Temperature diff") -> (x+y=w839:dbl)
            n795 = Subtract(x=w832, y="Temperature diff") -> (x-y=w838:dbl)
            n796 = Add(x=w831, y="Temperature diff") -> (x+y=w837:dbl)
            n797 = Subtract(x=w831, y="Temperature diff") -> (x-y=w836:dbl)
            n798 = In Range and Coerce(upper limit=w839, x=w841, lower limit=w838) -> (In Range?=w835:bool)  [unwired: 1 out]
            n799 = In Range and Coerce(upper limit=w837, x=w842, lower limit=w836) -> (In Range?=w834:bool)  [unwired: 1 out]
            n800 = And(x=w835, y=w834) -> (x .and. y?=w833:bool)
            n801 = case shown="True" w833 {
              frame False {
                n802 = property on="Accept & Save sample Temperature step 4" class="Bool (strict)"("DisabledEnum"=T19."Disabled" ("Disabled")) -> ()  [unwired: 2 in, 2 out]
                n803 = local write "Sample Temperature Calibration"(enum32{"True", "Fail"}."Fail" ("Sample Temperature Calibration  2")) -> ()
              }
              frame True {
                n804 = property on="Accept & Save sample Temperature step 4" class="Bool (strict)"("DisabledEnum"=T19."Enabled" ("Disabled")) -> ()  [unwired: 2 in, 2 out]
                n805 = local write "Sample Temperature Calibration"(enum32{"True", "Fail"}."True" ("Sample Temperature Calibration  2")) -> ()
              }
            }
          }
          frame #2 {
          }
          frame #3 {
          }
          frame #4 {
          }
          frame #5 {
          }
          frame #6 {
            # "CAL;END"
          }
          frame #7 {
          }
          frame #8 {
            # "CAL;END"
          }
          frame #9 {
            n806 = local write "Tab Control 4"(T14."Step 4" ("Tab Control 4")) -> ()
          }
        }
      }
      event "Accept & Save sample Temperature step 4": Value Change {
        n807 = event-data() -> ()  [unwired: 1 in, 6 out]
        n808 = stacked-sequence {
          frame #0 {
            n809 = local write "Due Write"("CAL;SAVE" ("Command")) -> ()
          }
          frame #1 {
            n810 = Wait (ms)(milliseconds to wait=u32 1000) -> ()  [unwired: 1 out]
          }
          frame #2 {
            n811 = local write "Due Write"("CAL;SAVE" ("Command")) -> ()
          }
          frame #3 {
            n812 = Wait (ms)(milliseconds to wait=u32 1000) -> ()  [unwired: 1 out]
          }
          frame #4 {
            n813 = local write "Due Write"("CAL;END" ("Command")) -> ()
          }
          frame #5 {
            n814 = Wait (ms)(milliseconds to wait=u32 1000) -> ()  [unwired: 1 out]
          }
          frame #6 {
            n815 = local write "Due Write"("CAL;END" ("Command")) -> ()
            n816 = local write "Temperature Selection"(T15."Default" ("Temperature Selection")) -> ()
            n817 = local write "Calibration Selection"(T10."Default" ("Calibration Selection")) -> ()
            n818 = local write "Tab Control 4"(T14."Main" ("Tab Control 4")) -> ()
            n819 = local write "Main Calibration Tab"(T9."Temperature" ("Main Calibration Tab")) -> ()
          }
          frame #7 {
            n820 = Get Date/Time In Seconds() -> (seconds since 1Jan1904=w861:timestamp)
            n821 = Format Into String(format string="%<%m/%d/%Y %I:%M:%S %p>T", w861) -> (resulting string=w859:string)  [unwired: 2 in, 1 out]
            n822 = local write "TEMPERATURE CALIBRATION"(w859) -> ()
          }
          frame #8 {
            n823 = local write "Save Button"(TRUE ("Save Button")) -> ()
            n824 = local write "Tab Control 4"(T14."Main" ("Tab Control 4")) -> ()
          }
        }
      }
      event "Accept & Save Air Temperature step 4": Value Change {
        n825 = event-data() -> ()  [unwired: 1 in, 6 out]
        n826 = stacked-sequence {
          frame #0 {
            n827 = local write "Due Write"("CAL;SAVE" ("Command")) -> ()
          }
          frame #1 {
            n828 = Wait (ms)(milliseconds to wait=u32 1000) -> ()  [unwired: 1 out]
          }
          frame #2 {
            n829 = local write "Due Write"("CAL;SAVE" ("Command")) -> ()
          }
          frame #3 {
            n830 = Wait (ms)(milliseconds to wait=u32 1000) -> ()  [unwired: 1 out]
          }
          frame #4 {
            n831 = local write "Due Write"("CAL;END" ("Command")) -> ()
          }
          frame #5 {
            n832 = Wait (ms)(milliseconds to wait=u32 1000) -> ()  [unwired: 1 out]
          }
          frame #6 {
            n833 = local write "Due Write"("CAL;END" ("Command")) -> ()
            n834 = local write "Tab Control 4"(T14."Main" ("Tab Control 4")) -> ()
            n835 = local write "Main Calibration Tab"(T9."Temperature" ("Main Calibration Tab")) -> ()
            n836 = local write "Temperature Selection"(T15."Default" ("Temperature Selection")) -> ()
            n837 = local write "Calibration Selection"(T10."Default" ("Calibration Selection")) -> ()
          }
          frame #7 {
            n838 = Get Date/Time In Seconds() -> (seconds since 1Jan1904=w877:timestamp)
            n839 = Format Into String(format string="%<%m/%d/%Y %I:%M:%S %p>T", w877) -> (resulting string=w876:string)  [unwired: 2 in, 1 out]
            n840 = local write "TEMPERATURE CALIBRATION"(w876) -> ()
          }
          frame #8 {
            n841 = local write "Tab Control 4"(T14."Main" ("Tab Control 4")) -> ()
            n842 = local write "Save Button"(TRUE ("Save Button")) -> ()
          }
        }
      }
      event "Temperature Continue Step 6": Value Change {
        n843 = event-data() -> ()  [unwired: 1 in, 6 out]
        n844 = stacked-sequence {
          frame #0 {
            n845 = stacked-sequence {
              frame #0 {
                n846 = Wait (ms)(milliseconds to wait=u32 1000) -> ()  [unwired: 1 out]
              }
              frame #1 {
              }
              frame #2 {
              }
              frame #3 {
                # "CAL;A1;<true_T>"
                n847 = local write "Due Write"("CAL;A1;60" ("Command")) -> ()
              }
              frame #4 {
                n848 = Wait (ms)(milliseconds to wait=u32 1000) -> ()  [unwired: 1 out]
              }
              frame #5 {
                # "CAL;A1;<true_T>"
                n849 = local write "Due Write"("CAL;A1;60" ("Command")) -> ()
              }
            }
          }
          frame #1 {
            n850 = local read "Sensor value"() -> (→"Air 60deg temp":dbl)
          }
          frame #2 {
          }
          frame #3 {
          }
          frame #4 {
          }
          frame #5 {
          }
          frame #6 {
            # "CAL;END"
          }
          frame #7 {
            w885 = 0.0 ("x")
            w886 = 60.0 ("x")
            n851 = local read "Temperature diff"() -> (w889:dbl)
            n852 = local read "Air 60deg temp"() -> (w888:dbl)
            n853 = local read "Air 0deg temp"() -> (w887:dbl)
            n854 = Add(x=w886, y=w889) -> (x+y=w896:dbl)
            n855 = Subtract(x=w886, y=w889) -> (x-y=w895:dbl)
            n856 = Add(x=w885, y=w889) -> (x+y=w894:dbl)
            n857 = Subtract(x=w885, y=w889) -> (x-y=w893:dbl)
            n858 = In Range and Coerce(upper limit=w896, x=w888, lower limit=w895) -> (In Range?=w892:bool)  [unwired: 1 out]
            n859 = In Range and Coerce(upper limit=w894, x=w887, lower limit=w893) -> (In Range?=w891:bool)  [unwired: 1 out]
            n860 = And(x=w892, y=w891) -> (x .and. y?=w890:bool)
            n861 = case shown="True" w890 {
              frame False {
                n862 = property on="Accept & Save Air Temperature step 4" class="Bool (strict)"("DisabledEnum"=T19."Disabled" ("Disabled")) -> ()  [unwired: 2 in, 2 out]
                n863 = local write "Air Temperature Calibration"(enum32{"True", "Fail"}."Fail" ("Sample Temperature Calibration  2")) -> ()
              }
              frame True {
                n864 = local write "Air Temperature Calibration"(enum32{"True", "Fail"}."True" ("Sample Temperature Calibration  2")) -> ()
                n865 = property on="Accept & Save Air Temperature step 4" class="Bool (strict)"("DisabledEnum"=T19."Enabled" ("Disabled")) -> ()  [unwired: 2 in, 2 out]
              }
            }
          }
          frame #8 {
            # "CAL;END"
          }
          frame #9 {
            n866 = local write "Tab Control 4"(T14."Air Step 4" ("Tab Control 4")) -> ()
          }
        }
      }
      event "Back Stroke step main temperature": Value Change {
        n867 = event-data() -> ()  [unwired: 1 in, 6 out]
        n868 = stacked-sequence {
          frame #0 {
            n869 = Wait (ms)(milliseconds to wait=u32 1000) -> ()  [unwired: 1 out]
          }
          frame #1 {
            # "CAL;END"
            n870 = local write "Due Write"("CAL;END" ("Command")) -> ()
          }
          frame #2 {
            n871 = Wait (ms)(milliseconds to wait=u32 1000) -> ()  [unwired: 1 out]
          }
          frame #3 {
            # "CAL;END"
            n872 = local write "Due Write"("CAL;END" ("Command")) -> ()
          }
          frame #4 {
            n873 = local write "Temperature Selection"(T15."Default" ("Temperature Selection")) -> ()
            n874 = local write "Calibration Selection"(T10."Default" ("Calibration Selection")) -> ()
            n875 = local write "Main Calibration Tab"(T9."Main" ("Main Calibration Tab")) -> ()
            n876 = local write "Tab Control 4"(T14."Main" ("Tab Control 4")) -> ()
          }
        }
      }
      event "TEMPERATURE STEP  Back 4", "TEMPERATURE STEP 1 Back 3", "TEMPERATURE STEP  Back 3", "TEMPERATURE STEP 1 Back 2", "Back Air TEMPERATURE Step 4", "Back SAMPLE TEMPERATURE Step 4": Value Change {
        # "Back Stroke step main temperature"
        n877 = event-data() -> ()  [unwired: 1 in, 6 out]
        n878 = stacked-sequence {
          frame #0 {
            n879 = Wait (ms)(milliseconds to wait=u32 1000) -> ()  [unwired: 1 out]
          }
          frame #1 {
            # "CAL;END"
            n880 = local write "Due Write"("CAL;END" ("Command")) -> ()
          }
          frame #2 {
            n881 = Wait (ms)(milliseconds to wait=u32 1000) -> ()  [unwired: 1 out]
          }
          frame #3 {
            # "CAL;END"
            n882 = local write "Due Write"("CAL;END" ("Command")) -> ()
          }
          frame #4 {
            # "TEMPERATURE STEP  Back 4"
            n883 = local write "Main Calibration Tab"(T9."Temperature" ("Main Calibration Tab")) -> ()
            n884 = local write "Temperature Selection"(T15."Default" ("Temperature Selection")) -> ()
            n885 = local write "Tab Control 4"(T14."Main" ("Tab Control 4")) -> ()
            n886 = local write "Calibration Selection"(T10."Default" ("Calibration Selection")) -> ()
          }
        }
      }
      event "FF BACK", "FF BACK 2", "FF BACK 3", "FF BACK 4", "FF BACK 5", "FF BACK 6": Value Change {
        n887 = event-data() -> ()  [unwired: 1 in, 6 out]
        n888 = stacked-sequence {
          frame #0 {
            n889 = Wait (ms)(milliseconds to wait=u32 1000) -> ()  [unwired: 1 out]
          }
          frame #1 {
            n890 = local write "Due Write"("VC;0") -> ()
          }
          frame #2 {
            n891 = Wait (ms)(milliseconds to wait=u32 1000) -> ()  [unwired: 1 out]
          }
          frame #3 {
            n892 = local write "Due Write"("VC;0") -> ()
          }
          frame #4 {
            w922 = FALSE
            n893 = local write "FF BACK 2"(w922) -> ()
            n894 = local write "FF BACK 3"(w922) -> ()
            n895 = local write "FF BACK 4"(w922) -> ()
            n896 = local write "FF BACK 5"(w922) -> ()
            n897 = local write "FF BACK 6"(w922) -> ()
            n898 = local write "FF BACK"(w922) -> ()
          }
          frame #5 {
            n899 = local write "Temperature Selection"(T15."Default" ("Temperature Selection")) -> ()
            n900 = local write "Calibration Selection"(T10."Default" ("Calibration Selection")) -> ()
            n901 = local write "Friction Force Tab"(T13."Page 1" ("Friction Force Tab")) -> ()
            n902 = local write "Main Calibration Tab"(T9."Main" ("Main Calibration Tab")) -> ()
